vi "coagBuffer.vi"(4 "all coag in":dbl[](array[numeric]), 6 "command":T1=enum."read recent", 8 "error in (no error)":errorcluster, 10 "max array size":u16=5000 min=1, 11 "Coag dose":dbl) -> (0 "error out":errorcluster, 1 "all coag out":dbl[](array[numeric]), 3 "recent coag":dbl)   [LabVIEW 2015]
uses:
  Sensor buffer command.ctl
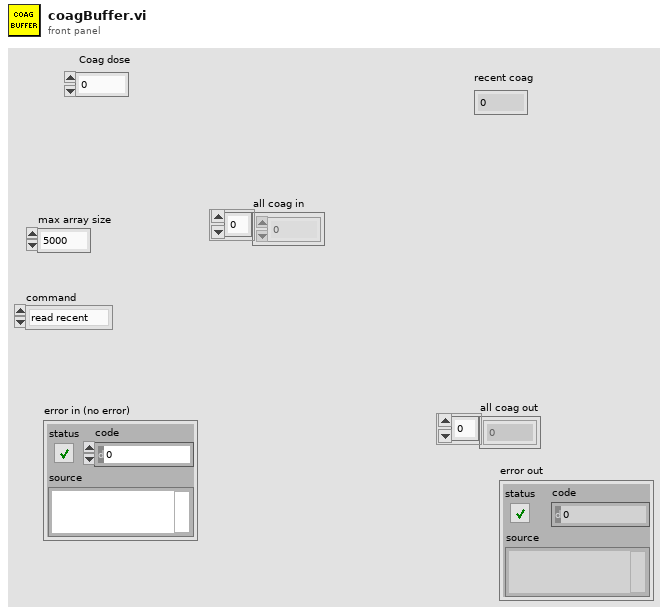
[diagram p1: front panel]
types:
  T1 = typedef "Sensor buffer command.ctl" = enum16{"set buffer size", "write", "refill buffer", "read recent", "read all", "clear"}
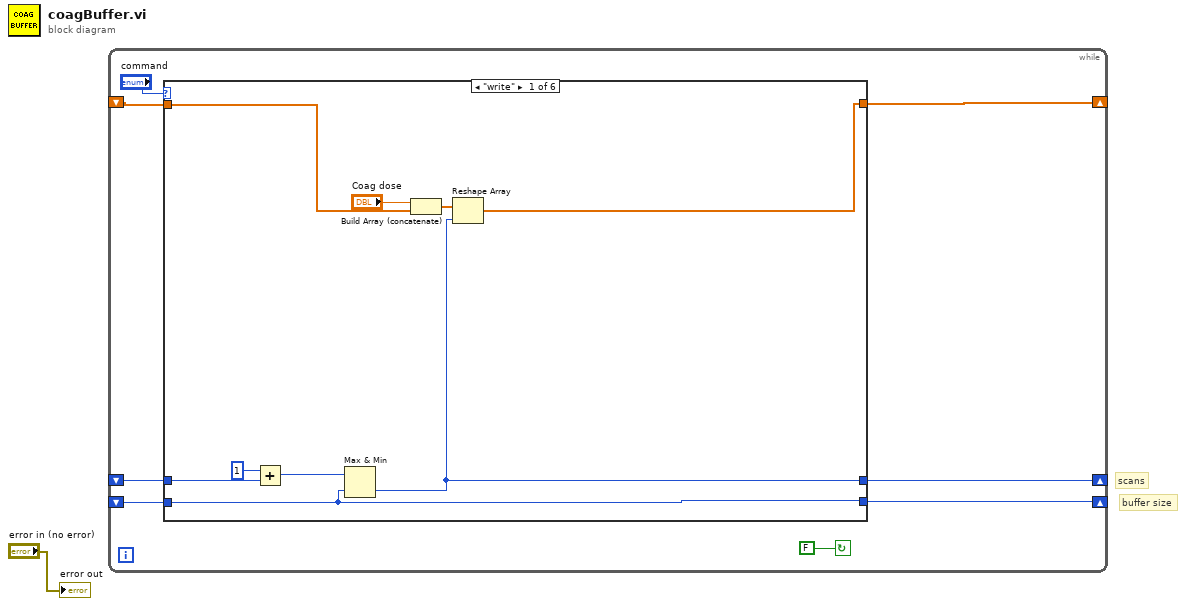
[diagram p0: block diagram]
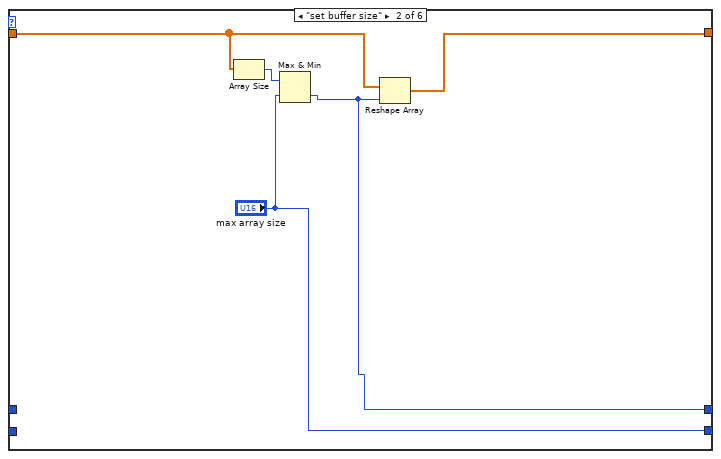
[diagram p2: hidden frame]
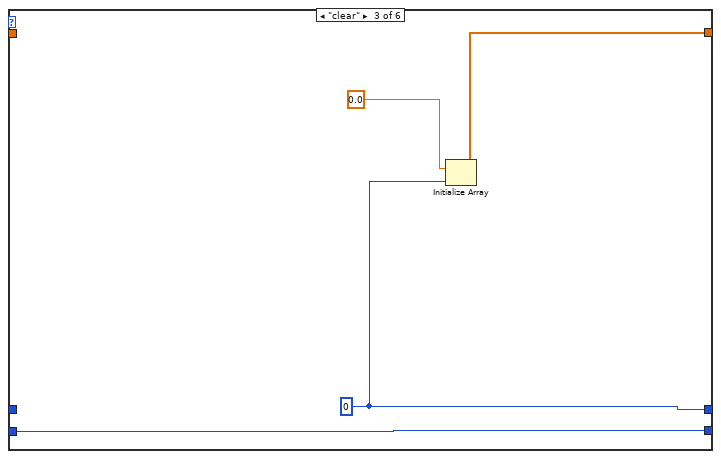
[diagram p3: hidden frame]
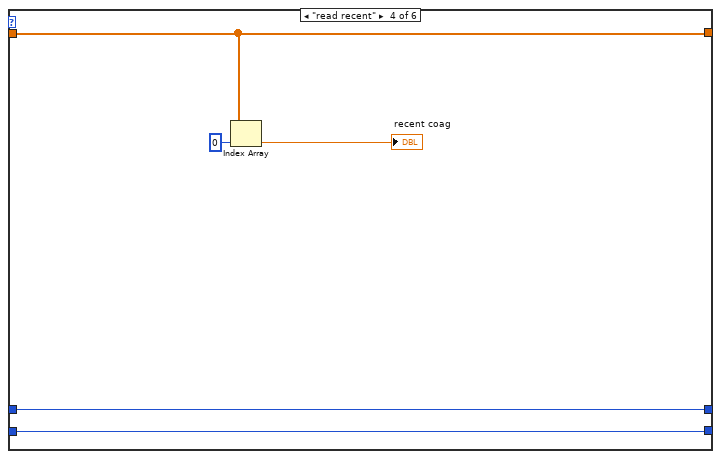
[diagram p4: hidden frame]
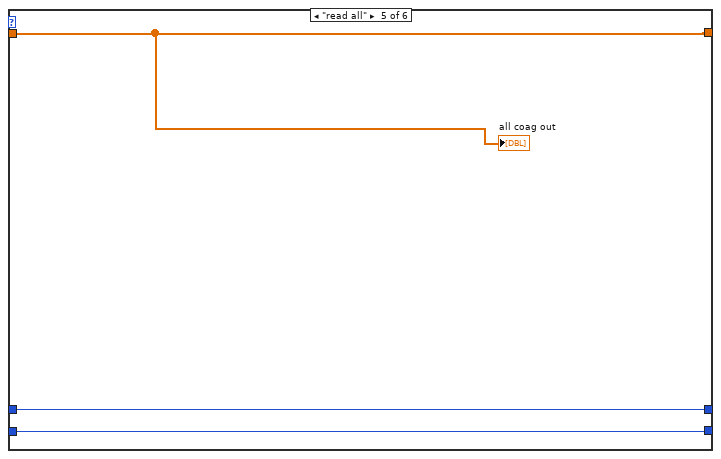
[diagram p5: hidden frame]
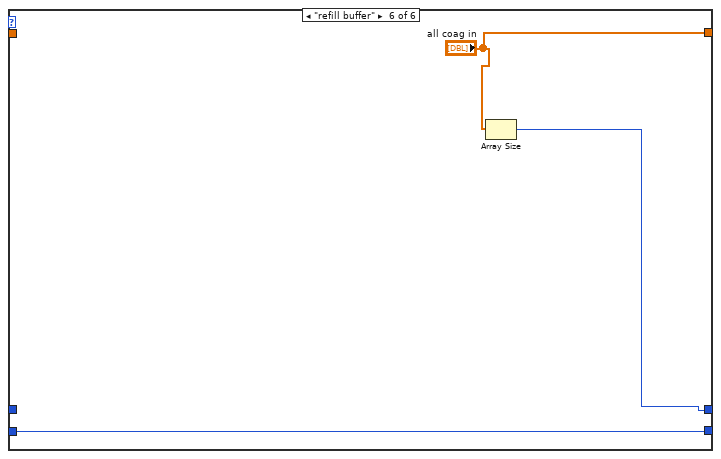
[diagram p6: hidden frame]
diagram:
  # "buffer size"
  # "scans"
  n1 = while {
    shift-right: [w8] -> _
    shift-left: _ -> [w7]
    shift-right: [w6] -> _
    shift-left: _ -> [w5]
    shift-right: [w2] -> _
    shift-left: _ -> [w3]
    stop <- FALSE continue-if-true
    n2 = case shown="\"write\"" "command" {
      tunnel: [w15 w23 w27 w32 w33 "all coag in"] -> w8
      tunnel: w7 -> [w17 w22 _ w32 w33 _]
      tunnel: [w11 "max array size" w26 w30 w35 w38] -> w6
      tunnel: w5 -> [w11 _ w26 w30 w35 w38]
      tunnel: w3 -> [w16 _ _ w29 w34 _]
      tunnel: [w10 w19 w24 w29 w34 w36] -> w2
      frame "write" {
        n3 = Add(x=1, y=w16) -> (x+y=w13:i32)
        n4 = Max & Min(x=w13, y=w11) -> (min(x,y)=w10:i32)  [unwired: 1 out]
        n5 = Build Array (concatenate)("Coag dose", w17) -> (w14:dbl[])
        n6 = Reshape Array(w14, w10) -> (w15:dbl[])
      }
      frame "set buffer size" {
        n7 = Array Size(array=w22) -> (size(s)=w21:i32)
        n8 = Max & Min(x=w21, y="max array size") -> (min(x,y)=w19:i32)  [unwired: 1 out]
        n9 = Reshape Array(w22, w19) -> (w23:dbl[])
      }
      frame "clear" {
        w24 = 0
        n10 = Initialize Array(0.0, w24) -> (w27:dbl[])
      }
      frame "read recent" {
        n11 = Index Array(array=w32, index=0) -> (element=→"recent coag":dbl)
      }
      frame "read all" {
        "all coag out" <- w33
      }
      frame "refill buffer" {
        n12 = Array Size(array="all coag in") -> (size(s)=w36:i32)
      }
    }
  }
  "error out" <- "error in (no error)"
